vi "CombineMode.vi"(10 "Obstacle Angle":dbl, 11 "Output to Goal in":T1) -> (3 "Output to Goal out":T1)   [LabVIEW 2016]
uses:
  <vilib>/Analysis/coordinate.llb/Angle Range (Degree).ctl
  <vilib>/Analysis/coordinate.llb/Angle Units.ctl
  <vilib>/Analysis/coordinate.llb/Wrap Angle (scalar).vi
  <vilib>/Analysis/NI_AAL_Angle.lvlib
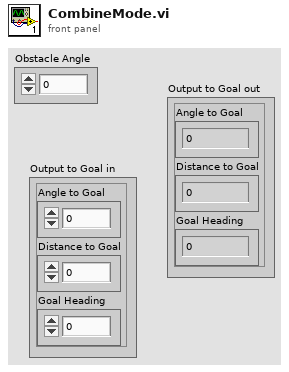
[diagram p1: front panel]
types:
  T1 = cluster{"Angle to Goal":dbl, "Distance to Goal":sgl, "Goal Heading":sgl}
  T2 = typedef "NI_AAL_Angle.lvlib/Angle Units.ctl" = i32
  T3 = typedef "NI_AAL_Angle.lvlib/Angle Range (Degree).ctl" = u16
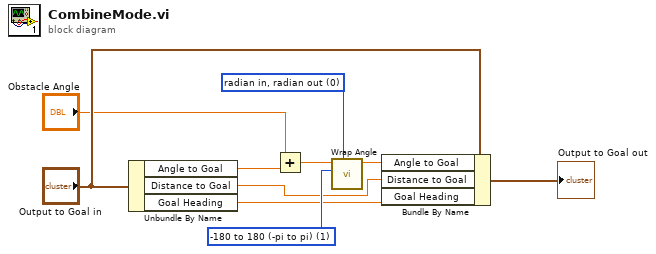
[diagram p0: block diagram]
diagram:
  w5 = T2 0 items=["radian in, radian out", "radian in, degree out", "degree in, degree out", "degree in, radian out"] ("angle units")
  w6 = T3 1 items=["none", "-180 to 180 (-pi to pi)", "0 to 360 (0 to 2pi)"] ("angle range")
  n1 = Unbundle By Name("Output to Goal in") -> ("Angle to Goal"=w8:dbl, "Distance to Goal"=w3:sgl, "Goal Heading"=w2:sgl)
  n2 = Add(x="Obstacle Angle", y=w8) -> (x+y=w7:dbl)
  n3 = call-poly <vilib>:"Wrap Angle.vi"("angle units"=w5, "angle range"=w6, "angle in"=w7) -> ("angle out"=w4:dbl)  [unwired: 7 in, 1 out]
  n4 = Bundle By Name(cluster="Output to Goal in", "Angle to Goal"=w4, "Distance to Goal"=w3, "Goal Heading"=w2) -> (→"Output to Goal out":T1)
